vi "Toggle Button.vi"(8 "starting state":bool, 11 "toggle button":bool) -> (3 "button toggled value":bool)   [LabVIEW 2014]
panel:
  in  "toggled state":bool
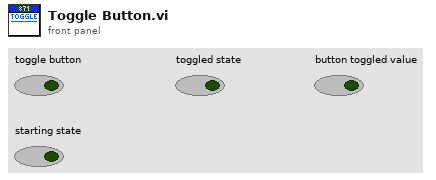
[diagram p1: front panel]
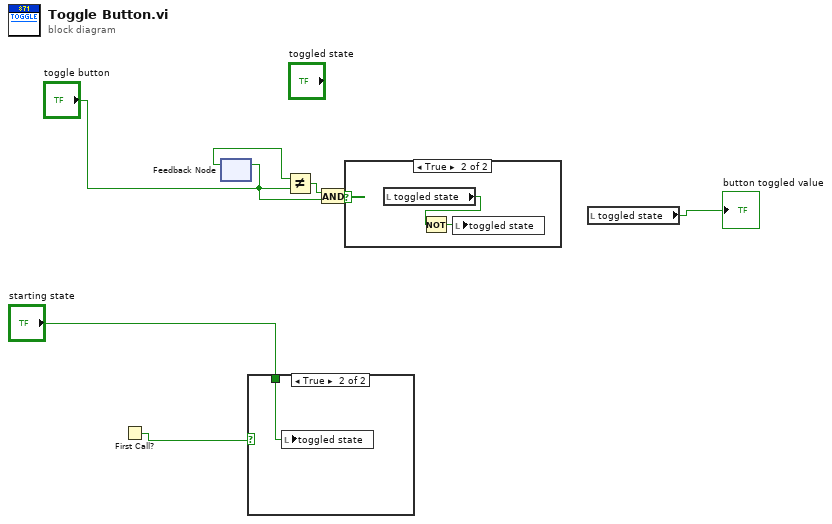
[diagram p0: block diagram]
diagram:
  n1 = First Call?() -> (First Call?: T/F=w3:bool)
  n2 = feedback #1() -> (w6:bool)  [unwired: 1 in]
  n3 = feedback-in #1("toggle button") -> ()
  n4 = case shown="True" w3 {
    tunnel: "starting state" -> [_ w8]
    frame False {
    }
    frame True {
      n5 = local write "toggled state"(w8) -> ()
    }
  }
  n6 = Not Equal?(x=w6, y="toggle button") -> (x != y?=w5:bool)
  n7 = And(x=w5, y="toggle button") -> (x .and. y?=w7:bool)
  n8 = case shown="True" w7 {
    frame False {
    }
    frame True {
      n9 = local read "toggled state"() -> (w10:bool)
      n10 = Not(x=w10) -> (.not. x?=w9:bool)
      n11 = local write "toggled state"(w9) -> ()
    }
  }
  n12 = local read "toggled state"() -> (→"button toggled value":bool)
